vi "功能计算_何 左.vi"(8 "截取%":i32, 9 "索引":i32=17, 10 "扭矩数组":dbl[](array[numeric])) -> (0 "扭差":dbl format="%#.2f", 1 "平均扭矩":dbl format="%#.2f", 2 "最小扭矩":dbl, 3 "峰值扭矩":dbl format="%#.2f")   [LabVIEW 2013]
panel:
  out "大小":i32
  out "第一个子数组":dbl[](array[numeric])
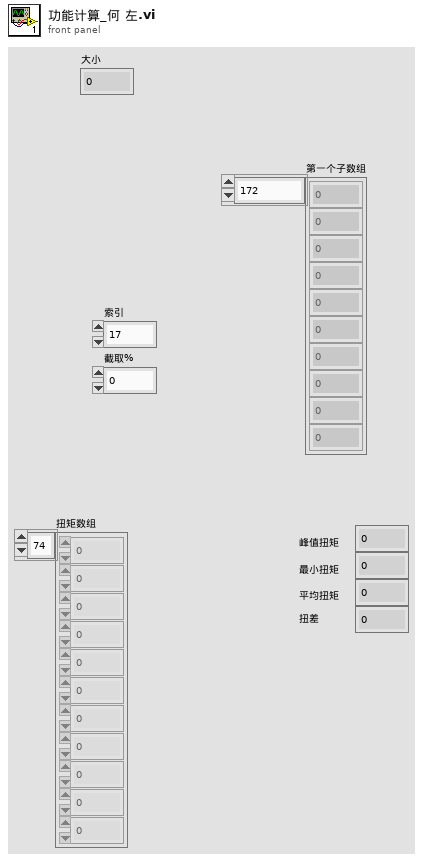
[diagram p1: front panel]
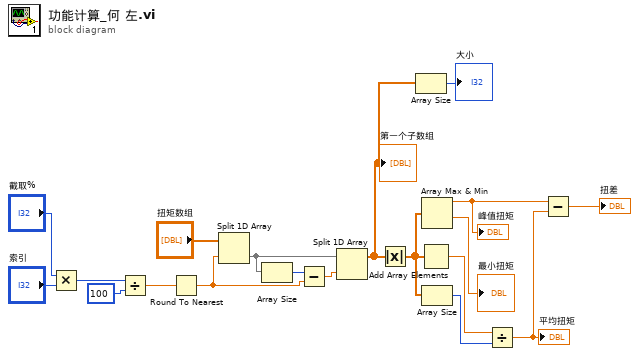
[diagram p0: block diagram]
diagram:
  n1 = Multiply(x="截取%", y="索引") -> (x*y=w4:i32)
  n2 = Divide(x=w4, y=100) -> (x/y=w5:dbl)
  n3 = Round To Nearest(number=w5) -> (nearest integer value=w6:dbl)
  n4 = Split 1D Array(array="扭矩数组", index=w6) -> (second subarray=w12:dbl[])  [unwired: 1 out]
  n5 = Array Size(array=w12) -> (size(s)=w11:i32)
  n6 = Subtract(x=w11, y=w6) -> (x-y=w10:dbl)
  n7 = Split 1D Array(array=w12, index=w10) -> (first subarray=w2:dbl[])  [unwired: 1 out]
  "第一个子数组" <- w2
  n8 = Absolute Value(x=w2) -> (abs(x)=w17:dbl[])
  n9 = Array Size(array=w2) -> (size(s)=→"大小":i32)
  n10 = Add Array Elements(numeric array=w17) -> (sum=w18:dbl)
  n11 = Array Max & Min(array=w17) -> (max value=w15:dbl, min value=→"最小扭矩":dbl)  [unwired: 2 out]
  "峰值扭矩" <- w15
  n12 = Array Size(array=w17) -> (size(s)=w16:i32)
  n13 = Divide(x=w18, y=w16) -> (x/y=w14:dbl)
  "平均扭矩" <- w14
  n14 = Subtract(x=w15, y=w14) -> (x-y=→"扭差":dbl)
